vi "SSL Detection Frame Simple Estimator Cameras VelCmd.vi"(0 "Lado":enum16{"Esquerdo", "Direito"}(ring)=enum."Direito" caption="Enum", 4 "IA State Input":T5={"our_robots"=[], "enemy_robots"=[], "balls"=[], "geometry"={"line_width"=0, "field_length"=0, "field_width"=0, "boundary_width"=0, "referee_width"=0, "goal_width"=0, "goal_depth"=0, "goal_wall_width"=0, "center_circle_radius"=0, "defense_radius"=0, "defense_stretch"=0, "free_kick_from_defense_dist"=0, "penalty_spot_from_field_line_dist"=0, "penalty_line_from_spot_dist"=0}, "IA Judge"={"stage"="", "command"="", "our_goalie_id"=0.0, "enemy_goalie_id"=0.0, "command enum"=enum."Halt", "Time"=enum."Azul"}, "Received Timestamp"=timestamp(0 s since 1904-01-01), "Events"={"Touch"=FALSE, "Ball out"=FALSE, "id touch"=0.0, "Ball out of \nVision"=FALSE, "Ball inside \nGoalie area"=FALSE, "Robot not responding"=FALSE, "Robots responding status"=[1.0, 1.0, 1.0, 1.0, 1.0, 1.0], "Enemy Ball \nPossession"=FALSE, "Pass State"=FALSE, "id end of pass"=0.0, "Kick"=FALSE, "Id ini Possession"=0.0, "Ball Possesion"=FALSE, "Id Possesion"=0.0, "Direct Kick"=FALSE, "2nd Strk Ativo"=FALSE}}, 5 "Estimador":T16, 6 "Time":enum16{"Azul", "Amarelo"}(ring) caption="Enum", 7 "Enable":bool, 8 "ignora esquerda?":bool=TRUE, 9 "ignora lado?":bool=TRUE, 10 "Field Size":T17, 11 "Detection Frame":T1 {"robots_blue"."height" format="%+4.3f"; "robots_blue"."pixel_y" format="%+4.3f"; "robots_blue"."pixel_x" format="%+4.3f"; "robots_blue"."orientation" format="%+4.3f"; "robots_blue"."y" format="%+4.3f"; "robots_blue"."confidence" format="%4.3f"; "robots_blue"."x" format="%+4.3f"; "robots_yellow"."height" format="%+4.3f"; "robots_yellow"."pixel_y" format="%+4.3f"; "robots_yellow"."pixel_x" format="%+4.3f"; "robots_yellow"."orientation" format="%+4.3f"; "robots_yellow"."y" format="%+4.3f"; "robots_yellow"."confidence" format="%4.3f"; "robots_yellow"."x" format="%+4.3f"}) -> (1 "Frame Array":T1[](array[typedef]) {"robots_blue"."height" format="%+4.3f"; "robots_blue"."pixel_y" format="%+4.3f"; "robots_blue"."pixel_x" format="%+4.3f"; "robots_blue"."orientation" format="%+4.3f"; "robots_blue"."y" format="%+4.3f"; "robots_blue"."confidence" format="%4.3f"; "robots_blue"."x" format="%+4.3f"; "robots_yellow"."height" format="%+4.3f"; "robots_yellow"."pixel_y" format="%+4.3f"; "robots_yellow"."pixel_x" format="%+4.3f"; "robots_yellow"."orientation" format="%+4.3f"; "robots_yellow"."y" format="%+4.3f"; "robots_yellow"."confidence" format="%4.3f"; "robots_yellow"."x" format="%+4.3f"}, 2 "Field Size Out":T17, 3 "Detection Frame Out":T1 {"robots_blue"."height" format="%+4.3f"; "robots_blue"."pixel_y" format="%+4.3f"; "robots_blue"."pixel_x" format="%+4.3f"; "robots_blue"."orientation" format="%+4.3f"; "robots_blue"."y" format="%+4.3f"; "robots_blue"."confidence" format="%4.3f"; "robots_blue"."x" format="%+4.3f"; "robots_yellow"."height" format="%+4.3f"; "robots_yellow"."pixel_y" format="%+4.3f"; "robots_yellow"."pixel_x" format="%+4.3f"; "robots_yellow"."orientation" format="%+4.3f"; "robots_yellow"."y" format="%+4.3f"; "robots_yellow"."confidence" format="%4.3f"; "robots_yellow"."x" format="%+4.3f"})   [LabVIEW 2018]
uses:
  SSL Detection Frame.ctl
  SSL Detection Robot.ctl
  <vilib>/Analysis/Matrix/Datatypes/RealMatrix.ctl
  SSL Detection Ball.ctl
  Filters/Estimadores.ctl
  Core/AI Input.ctl
  Core/AI Robot.ctl
  Intel/Functions Enum.ctl
  Intel/AttackerStates.ctl
  Path Planning/RRT/PathDests.ctl
  Path Planning/RRT/PathDest.ctl
  Core/AI Ball.ctl
  Core/Field Size.ctl
  Core/AI Judge.ctl
  Intel/Command Enum.ctl
  Events/Events.ctl
  <vilib>/Analysis/Matrix/NI_Matrix.lvlib
panel:
  out "output cluster":T1 {"robots_blue"."height" format="%+4.3f"; "robots_blue"."pixel_y" format="%+4.3f"; "robots_blue"."pixel_x" format="%+4.3f"; "robots_blue"."orientation" format="%+4.3f"; "robots_blue"."y" format="%+4.3f"; "robots_blue"."confidence" format="%4.3f"; "robots_blue"."x" format="%+4.3f"; "robots_yellow"."height" format="%+4.3f"; "robots_yellow"."pixel_y" format="%+4.3f"; "robots_yellow"."pixel_x" format="%+4.3f"; "robots_yellow"."orientation" format="%+4.3f"; "robots_yellow"."y" format="%+4.3f"; "robots_yellow"."confidence" format="%4.3f"; "robots_yellow"."x" format="%+4.3f"}
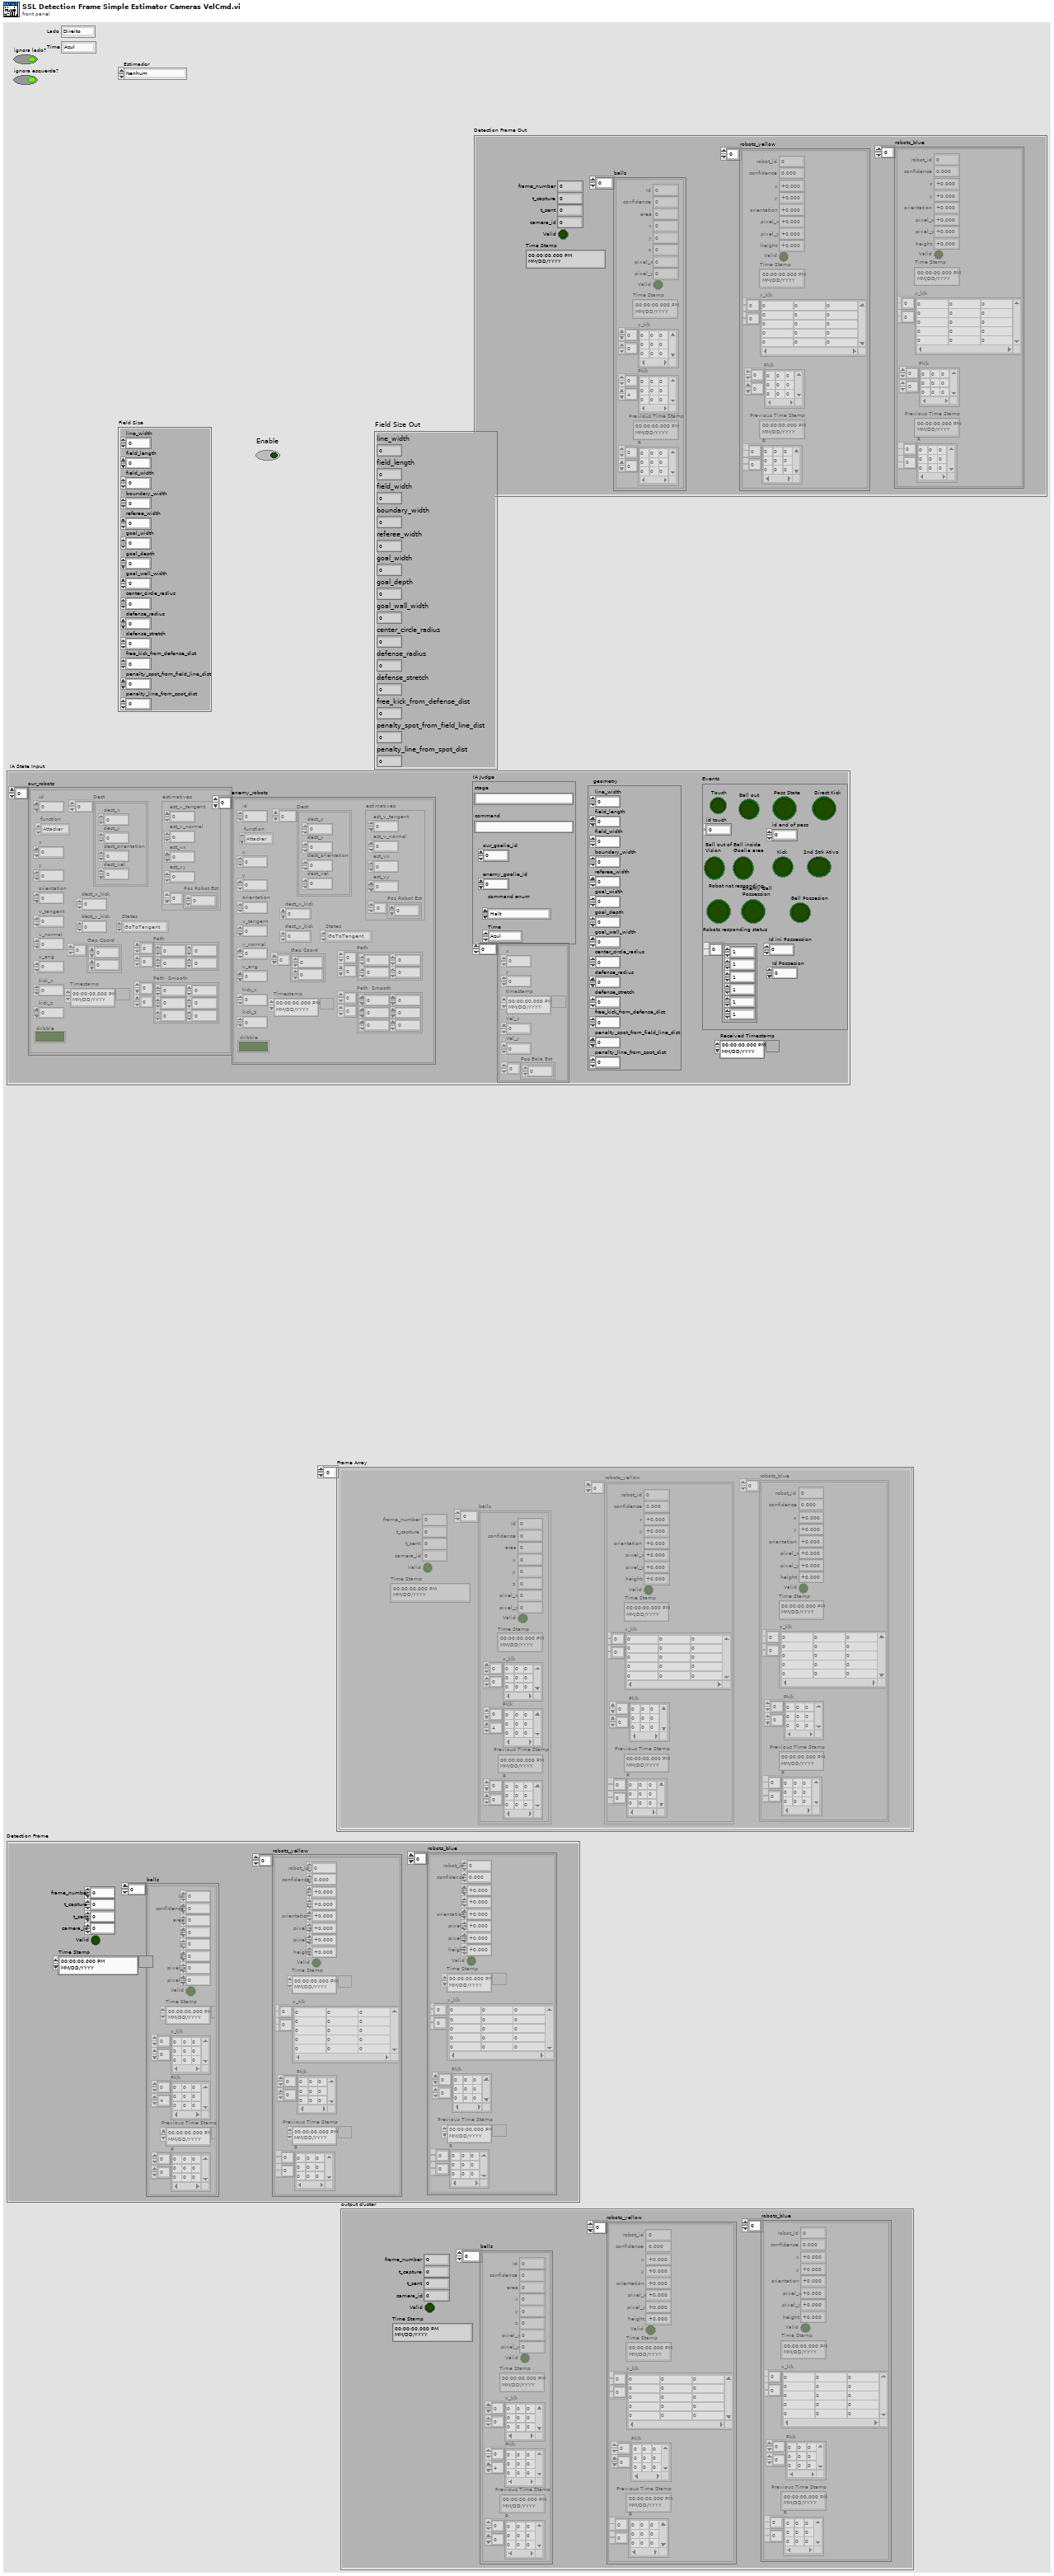
[diagram p1: front panel]
types:
  T1 = typedef "SSL Detection Frame.ctl" = cluster{"frame_number":u32, "t_capture":dbl, "t_sent":dbl, "camera_id":u32, "robots_yellow":T2[], "robots_blue":T2[], "balls":T4[], "Valid":bool, "Time Stamp":timestamp}
  T2 = typedef "SSL Detection Robot.ctl" = cluster{"x":sgl, "robot_id":u32, "confidence":sgl, "y":sgl, "orientation":sgl, "pixel_x":sgl, "pixel_y":sgl, "height":sgl, "Valid":bool, "Time Stamp":timestamp, "x_k|k":T3, "Pk|k":T3, "Previous Time Stamp":timestamp, "R":T3}
  T3 = typedef "NI_Matrix.lvlib/RealMatrix.ctl" = dbl[][]
  T4 = typedef "SSL Detection Ball.ctl" = cluster{"x":sgl, "area":u32, "confidence":sgl, "y":sgl, "z":sgl, "pixel_x":sgl, "pixel_y":sgl, "Valid":bool, "Time Stamp":timestamp, "x_k|k":T3, "Pk|k":T3, "Id":u32, "Previous Time Stamp":timestamp, "R":T3}
  T5 = typedef "AI Input.ctl" = cluster{"our_robots":T6[], "enemy_robots":T6[], "balls":T11[], "geometry":T12, "IA Judge":T13, "Received Timestamp":timestamp, "Events":T15}
  T6 = typedef "AI Robot.ctl" = cluster{"id":u32, "function":T7, "x":dbl, "y":dbl, "orientation":dbl, "v_tangent":dbl, "v_normal":dbl, "v_ang":dbl, "kick_x":dbl, "kick_z":dbl, "dribble":bool, "Timestamp":timestamp, "estimatives":cluster{"est_v_tangent":dbl, "est_v_normal":dbl, "est_vx":dbl, "est_vy":dbl, "Pos Robot Est":dbl[]}, "dest_x_kick":dbl, "dest_y_kick":dbl, "Gap Coord":dbl[], "States":T8, "Path ":dbl[][], "Path  Smooth":dbl[][], "Dest":T9}
  T7 = typedef "Functions Enum.ctl" = enum16{"2nd Striker", "Attacker", "Goalie", "Defender", "Striker", "Goto 0", "Dummy", "Kicker", "ZigZag 0", "ZigZag 1", "ZigZag 2", "ZigZag 3", "ZigZag 4", "ZigZag 5", "ZigZag 6", "ZigZag 7", "ZigZag 8", ""}
  T8 = typedef "AttackerStates.ctl" = enum16{"Pass", "GoToTangent", "BallGetting", "GoToKick", ""}
  T9 = typedef "PathDests.ctl" = T10[]
  T10 = typedef "PathDest.ctl" = cluster{"dest_x":dbl, "dest_y":dbl, "dest_orientation":dbl, "dest_vel":dbl}
  T11 = typedef "AI Ball.ctl" = cluster{"x":dbl, "y":dbl, "timestamp":timestamp, "Vel_x":dbl, "Vel_y":dbl, "Pos Bola Est":dbl[]}
  T12 = typedef "Field Size.ctl" = cluster{"line_width":u32, "field_length":u32, "field_width":u32, "boundary_width":u32, "referee_width":u32, "goal_width":u32, "goal_depth":u32, "goal_wall_width":u32, "center_circle_radius":u32, "defense_radius":u32, "defense_stretch":u32, "free_kick_from_defense_dist":u32, "penalty_spot_from_field_line_dist":u32, "penalty_line_from_spot_dist":u32}
  T13 = typedef "AI Judge.ctl" = cluster{"stage":string, "command":string, "our_goalie_id":dbl, "enemy_goalie_id":dbl, "command enum":T14, "Time":enum16{"Azul", "Amarelo"}}
  T14 = typedef "Command Enum.ctl" = enum16{"Halt", "Stop", "Force Start", "PKA Normal Start", "Prepare Kickoff Ally", "PKE Normal Start", "Prepare Kickoff Enemy", "Prepare Penalty Ally", "PPA Normal Start", "Prepare Penalty Enemy", "PPE Normal Start", "Direct Free Enemy", "Direct Free Ally", "Indirect Free Enemy", "Indirect Free Ally", "Timeout Enemy", "Timeout Ally", "Goal Enemy", "Goal Ally", "Ball Placement Enemy", "Ball Placement Ally", "Normal Half Time", "Extra Time Break", "Extra Half Time", "None", "Post Game"}
  T15 = typedef "Events.ctl" = cluster{"Touch":bool, "Ball out":bool, "id touch":dbl, "Ball out of \nVision":bool, "Ball inside \nGoalie area":bool, "Robot not responding":bool, "Robots responding status":dbl[], "Enemy Ball \nPossession":bool, "Pass State":bool, "id end of pass":dbl, "Kick":bool, "Id ini Possession":dbl, "Ball Possesion":bool, "Id Possesion":dbl, "Direct Kick":bool, "2nd Strk Ativo":bool}
  T16 = typedef "Estimadores.ctl" = enum16{"Nenhum", "Simples", "Kalman"}
  T17 = cluster{"line_width":u32, "field_length":u32, "field_width":u32, "boundary_width":u32, "referee_width":u32, "goal_width":u32, "goal_depth":u32, "goal_wall_width":u32, "center_circle_radius":u32, "defense_radius":u32, "defense_stretch":u32, "free_kick_from_defense_dist":u32, "penalty_spot_from_field_line_dist":u32, "penalty_line_from_spot_dist":u32}
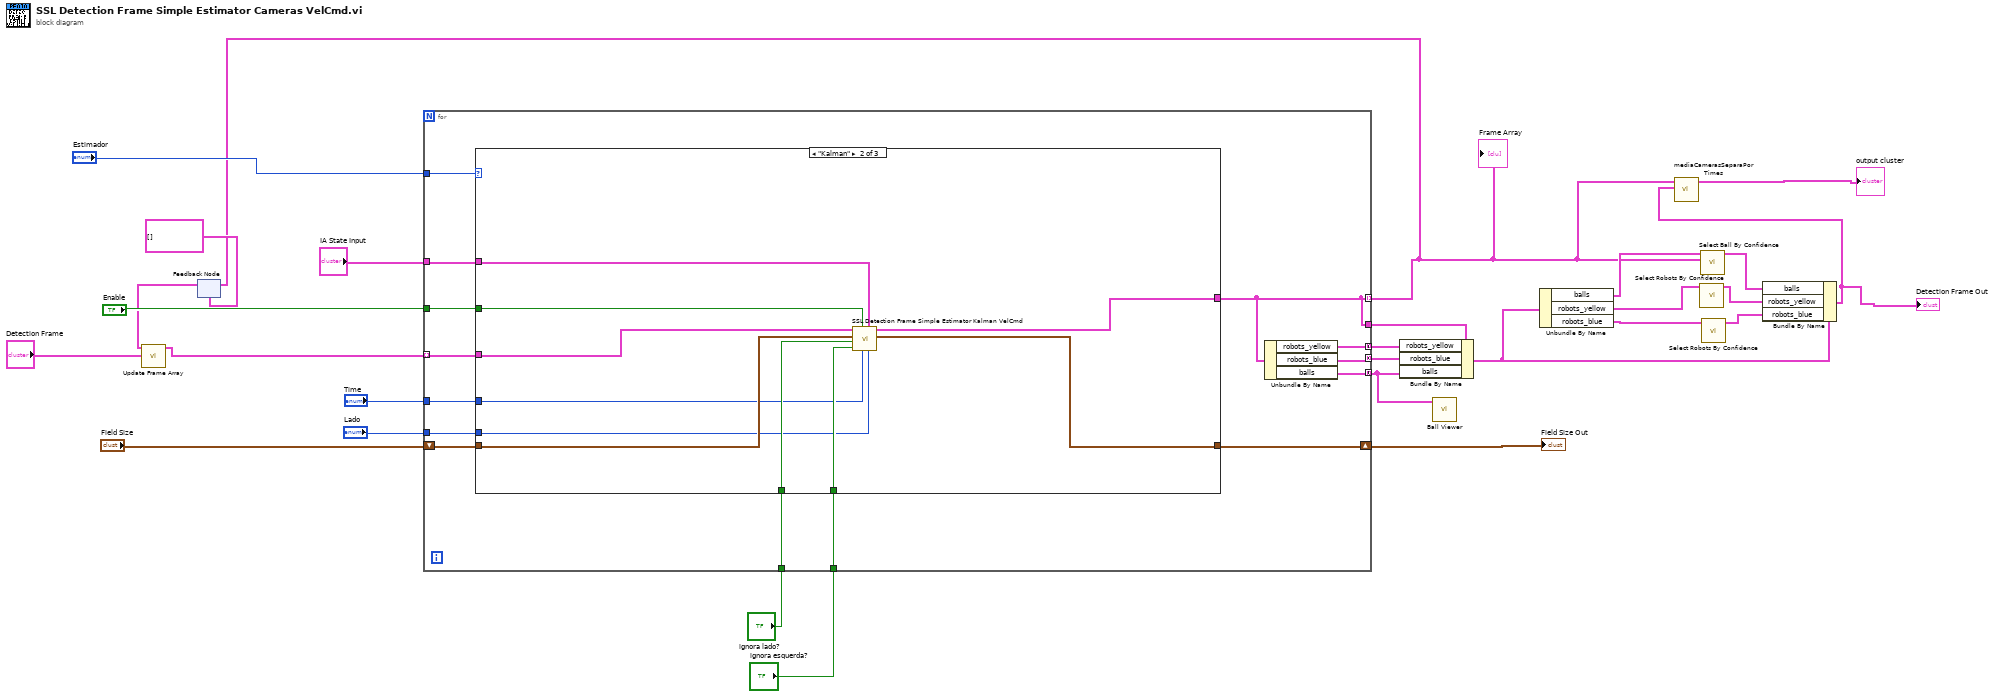
[diagram p0: block diagram]
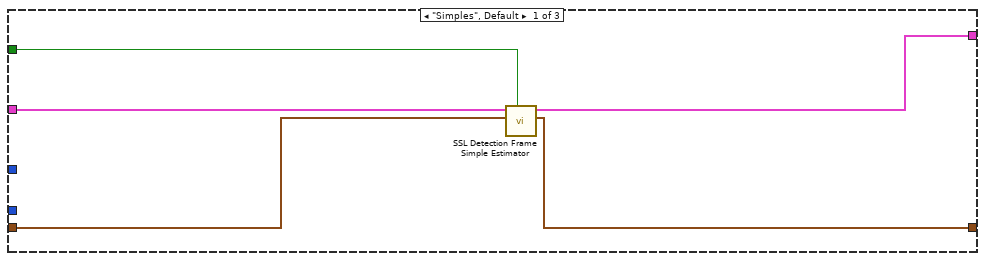
[diagram p2: hidden frame]
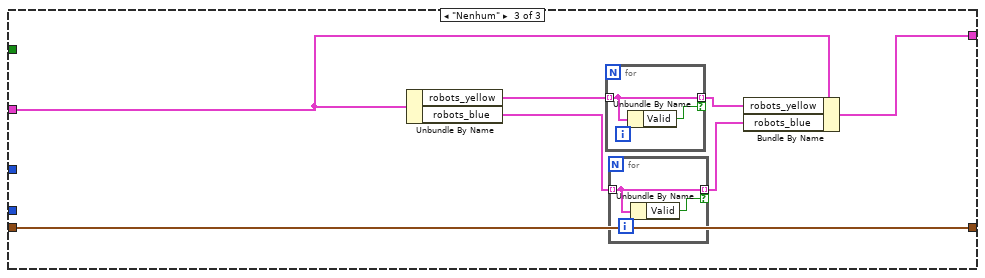
[diagram p3: hidden frame]
diagram:
  n1 = feedback #1(T1[] []) -> (w6:T1[])
  n2 = call "Update Frame Array.vi"("Detection Frame In"="Detection Frame", "Array Detection Frame In"=w6) -> ("Detection Frame In out"=w8:T1[])  [unwired: 9 in]
  n3 = for {
    tunnel: [w33] -> w4 mode=indexing
    tunnel: "Estimador" -> [w39]
    tunnel: "Enable" -> [w38]
    tunnel: w8 -> [w37] mode=indexing
    shift-right: [w40] -> w27
    shift-left: "Field Size" -> [w41]
    tunnel: [w36] -> w24 mode=concatenating
    tunnel: [w35] -> w23 mode=concatenating
    tunnel: [w34] -> w15 mode=concatenating
    tunnel: [w33] -> w25
    tunnel: "ignora lado?" -> [w32]
    tunnel: "ignora esquerda?" -> [w31]
    tunnel: "Time" -> [w30]
    tunnel: "IA State Input" -> [w29]
    tunnel: "Lado" -> [w28]
    n4 = case shown="\"Kalman\"" w39 {
      tunnel: [w42 w55 w59] -> w33
      tunnel: w37 -> [w46 w56 w61]
      tunnel: w38 -> [w45 w52 _]
      tunnel: w41 -> [w44 w54 w63]
      tunnel: [w43 w53 w63] -> w40
      tunnel: w32 -> [_ w51 _]
      tunnel: w31 -> [_ w50 _]
      tunnel: w30 -> [_ w49 _]
      tunnel: w29 -> [_ w48 _]
      tunnel: w28 -> [_ w47 _]
      frame "Simples", Default {
        n5 = call "SSL Detection Frame Simple Estimator.vi"("Enable"=w45, "Field Size"=w44, "Detection Frame In"=w46) -> ("Field Size Out"=w43:T17, "Detection Frame Out"=w42:T1)  [unwired: 7 in]
      }
      frame "Kalman" {
        n6 = call "SSL Detection Frame Simple Estimator Kalman VelCmd.vi"("Lado"=w47, "IA State Output"=w48, "Time"=w49, "Enable"=w52, "ignora esquerda?"=w50, "ignora lado?"=w51, "Field Size"=w54, "Detection Frame In"=w56) -> ("Field Size Out"=w53:T17, "Detection Frame Out"=w55:T1)  [unwired: 2 in]
      }
      frame "Nenhum" {
        n7 = Unbundle By Name(w61) -> ("robots_yellow"=w62:T2[], "robots_blue"=w58:T2[])
        n8 = for {
          tunnel: w62 -> [w67] mode=indexing
          tunnel: [w67] -> w60 mode=indexing if=w66
          n9 = Unbundle By Name(w67) -> ("Valid"=w66:bool)
        }
        n10 = for {
          tunnel: w58 -> [w65] mode=indexing
          tunnel: [w65] -> w57 mode=indexing if=w64
          n11 = Unbundle By Name(w65) -> ("Valid"=w64:bool)
        }
        n12 = Bundle By Name(cluster=w61, "robots_yellow"=w60, "robots_blue"=w57) -> (w59:T1)
      }
    }
    n13 = Unbundle By Name(w33) -> ("robots_yellow"=w36:T2[], "robots_blue"=w35:T2[], "balls"=w34:T4[])
  }
  "Field Size Out" <- w27
  "Frame Array" <- w4
  n14 = feedback-in #1(w4) -> ()
  n15 = Bundle By Name(cluster=w25, "robots_yellow"=w24, "robots_blue"=w23, "balls"=w15) -> (w3:T1)
  n16 = call "Ball Viewer.vi"("balls"=w15) -> ()  [unwired: 11 in]
  n17 = Unbundle By Name(w3) -> ("balls"=w14:T4[], "robots_yellow"=w19:T2[], "robots_blue"=w22:T2[])
  n18 = call "Select Robots By Confidence.vi"("robots_blue"=w19) -> ("Array"=w18:T2[])  [unwired: 10 in]
  n19 = call "Select Ball By Confidence.vi"("Array"=w4, "balls"=w14) -> ("balls out"=w13:T4[])  [unwired: 9 in]
  n20 = call "Select Robots By Confidence.vi"("robots_blue"=w22) -> ("Array"=w21:T2[])  [unwired: 10 in]
  n21 = Bundle By Name(cluster=w3, "balls"=w13, "robots_yellow"=w18, "robots_blue"=w21) -> (w1:T1)
  "Detection Frame Out" <- w1
  n22 = call "mediaCamerasSeparaPorTimes.vi"("input cluster 2"=w1, "Frame Array"=w4) -> ("output cluster"=→"output cluster":T1)  [unwired: 7 in]
